vi "portinarisat_monitoreo.vi"() -> ()   [LabVIEW 2024]
uses:
  <vilib>/Instr/_visa.llb/VISA Configure Serial Port (Instr).vi
panel:
  out "?":dbl
  out "?":dbl
  out "?":dbl
  out "?":dbl
  out "?":dbl
  out "?":dbl
  out "?":dbl
  out "?":dbl
  out "?":dbl
  out "Trama original":string
  in  "Baudios":u32=9600
  in  "Puerto serial":refnum<visa-resource-name>
  in  "stop":bool
  out "Tiempo (s)":dbl
  out "Altitud":dbl
  out "Altitud (m)":dbl(slide) scale=0.0..500.0
  out "Altitud":i32(graph)
  out "Temperatura":i32(graph)
  out "Presión":i32(graph)
  out "CO2":i32(graph)
  out "CO2":dbl
  out "CO2 (ppm)":dbl(knob) scale=300.0..1000.0
  out "Temperatura":dbl
  out "Presiòn":dbl
  out "Velocidad":dbl
  out "G Eje Z":dbl(slide) caption="Eje Z" scale=-250.0..250.0
  out "G Eje Y":dbl(slide) caption="Eje Y" scale=-250.0..250.0
  out "G Eje X":dbl(slide) caption="Eje X" scale=-250.0..250.0
  out "CM Eje Z":dbl(slide) caption="Eje Z" scale=-60.0..60.0
  out "CM Eje Y":dbl(slide) caption="Eje Y" scale=-60.0..60.0
  out "CM Eje X":dbl(slide) caption="Eje X" scale=-60.0..60.0
  out "A Eje Z":dbl(slide) caption="Eje Z" scale=-20.0..20.0
  out "A Eje Y":dbl(slide) caption="Eje Y" scale=-20.0..20.0
  out "A Eje X":dbl(slide) caption="Eje X" scale=-20.0..20.0
  out "Velocidad (m/s)":dbl(knob) scale=-10.0..50.0
  out "Presión (kPa)":dbl(knob) scale=60.0..110.0
  out "Temperatura (°C)":dbl(slide) scale=-10.0..50.0
  # "Aceleración (m/s^2)"
  # "Campo magnético (µT)"
  # "Velocidad angular (°/s)"
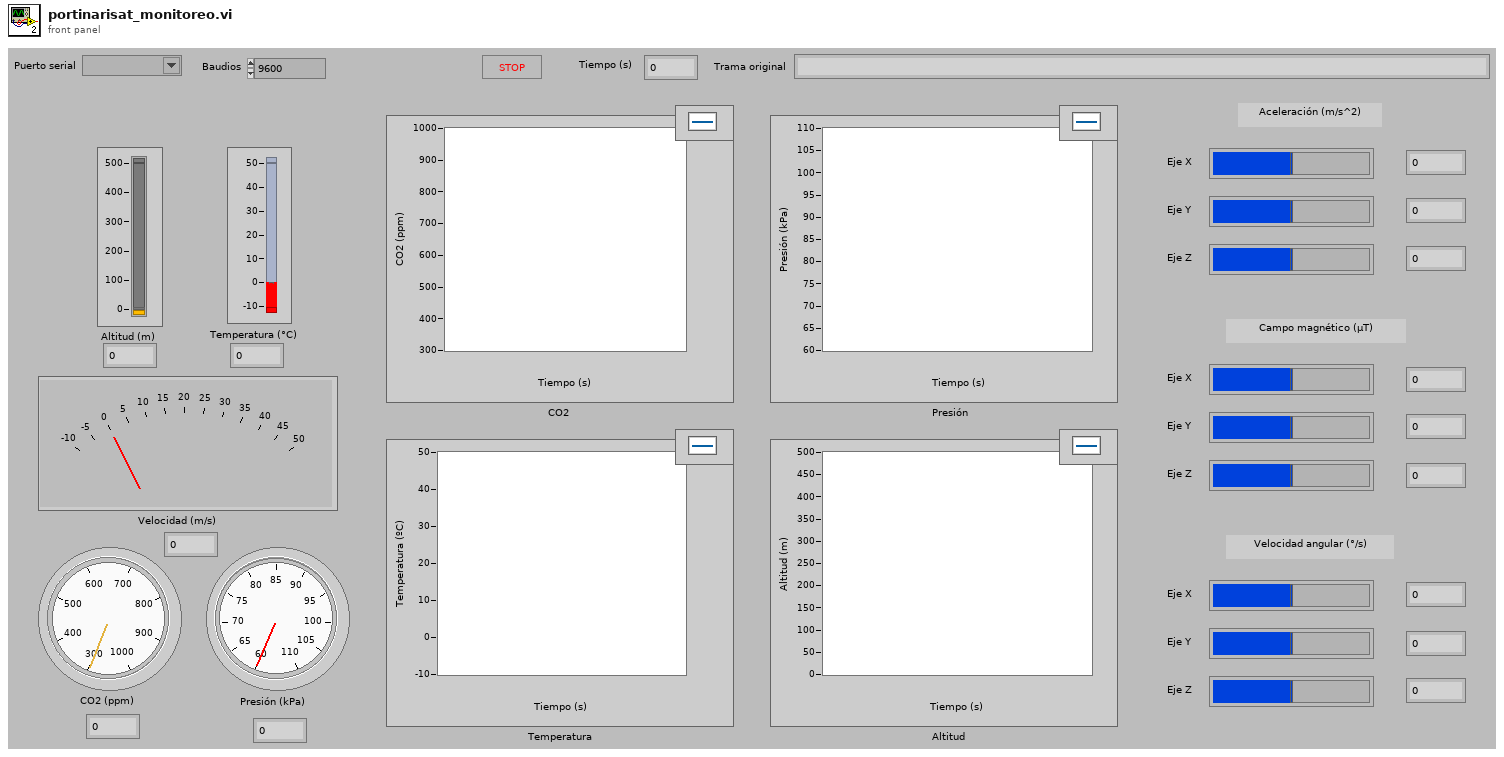
[diagram p1: front panel]
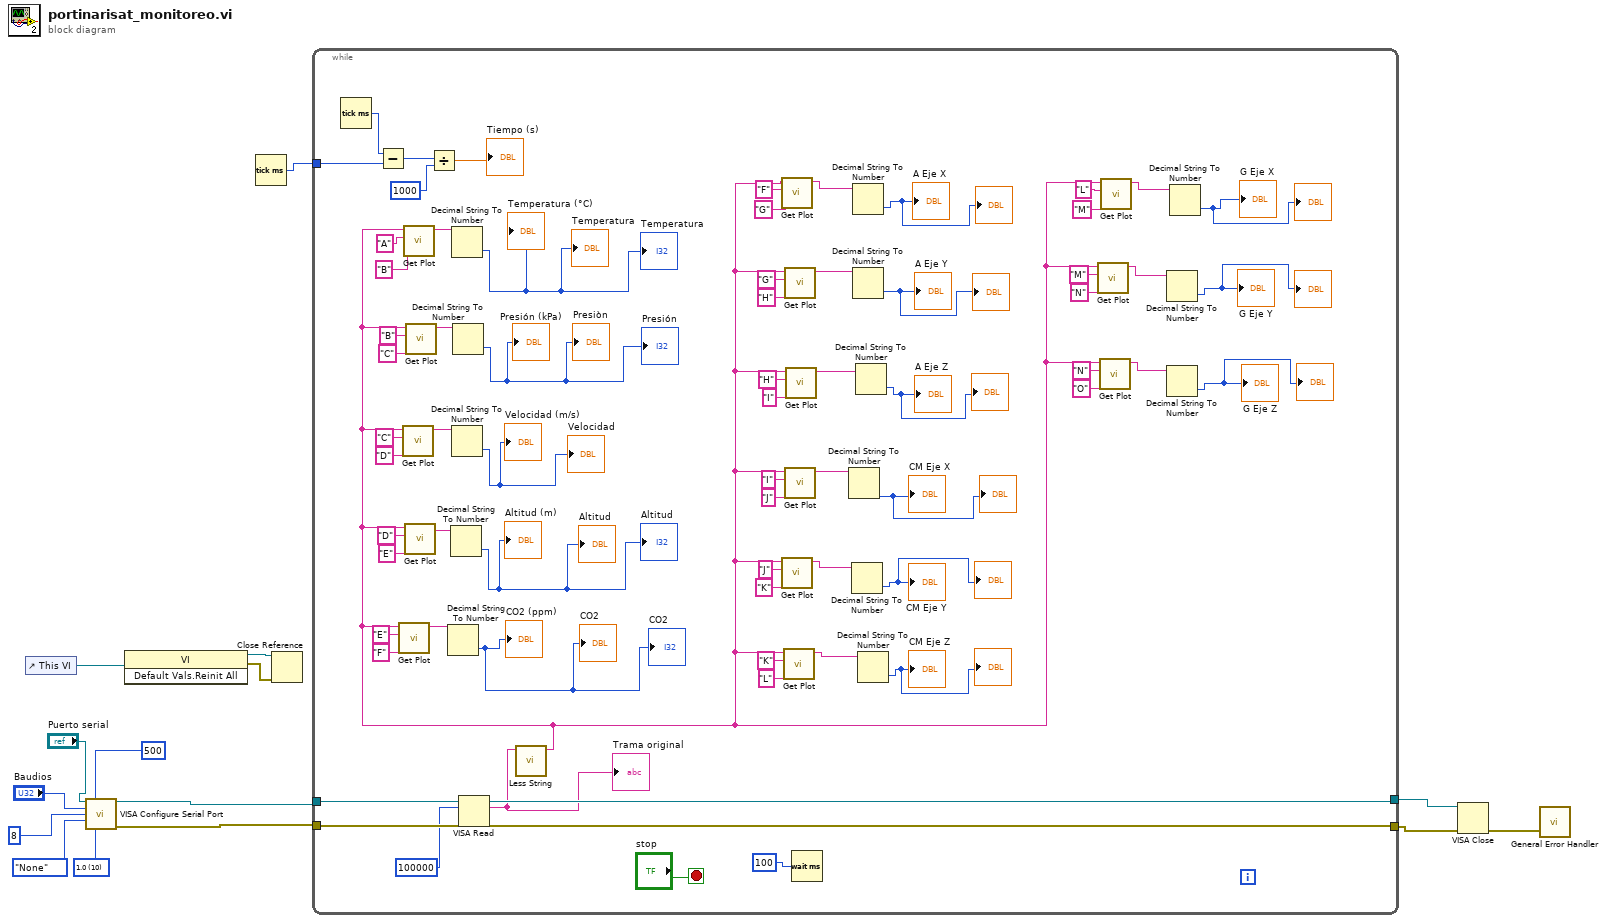
[diagram p0: block diagram]
diagram:
  w2 = u16 10 items=["1.0"=10, "1.5"=15, "2.0"=20] ("stop bits (10: 1 bit)")
  n1 = control-ref of="This VI"() -> (w8:refnum<vi>)
  n2 = call-poly "VISA Configure Serial Port"("VISA resource name"="Puerto serial", "timeout (10sec)"=u32 500, "baud rate (9600)"="Baudios", "data bits (8)"=u16 8, "parity (0:none)"=enum16{"None", "Odd", "Even", "Mark", "Space"}."None", "stop bits (10: 1 bit)"=w2) -> ("VISA resource name out"=w6:refnum<visa-resource-name>, "error out"=w5:errorcluster)  [unwired: 8 in]
  n3 = invoke class="VI" method="Default Vals.Reinit All"(reference=w8) -> (reference out=w9:refnum<vi>, error out=w7:errorcluster)  [unwired: 2 in, 1 out]
  n4 = Tick Count (ms)() -> (millisecond timer value=w11:u32)
  n5 = Close Reference(reference=w9, error in (no error)=w7) -> ()  [unwired: 1 out]
  n6 = while {
    tunnel: w6 -> [w28]
    tunnel: [w85] -> w13
    tunnel: [w83] -> w12
    tunnel: w11 -> [w33]
    tunnel: w5 -> [w29]
    stop <- "stop" stop-if-true
    n7 = Tick Count (ms)() -> (millisecond timer value=w34:u32)
    n8 = Subtract(x=w34, y=w33) -> (x-y=w32:u32)
    n9 = Divide(x=w32, y=u32 1000) -> (x/y=→"Tiempo (s)":dbl)
    n10 = VISA Read(VISA resource name=w28, byte count=u32 100000, error in (no error)=w29) -> (VISA resource name out=w85:refnum<visa-resource-name>, read buffer=w30:string, error out=w83:errorcluster)  [unwired: 1 out]
    "Trama original" <- w30
    n11 = call "Less String.vi"("Input String"=w30) -> ("Out String"=w60:string)  [unwired: 10 in]
    n12 = call "Get Plot.vi"("Stop"="F", "Start"="E", "Input String"=w60) -> ("Out String"=w47:string)  [unwired: 8 in]
    n13 = call "Get Plot.vi"("Stop"="D", "Start"="C", "Input String"=w60) -> ("Out String"=w50:string)  [unwired: 8 in]
    n14 = call "Get Plot.vi"("Stop"="B", "Start"="A", "Input String"=w60) -> ("Out String"=w53:string)  [unwired: 8 in]
    n15 = call "Get Plot.vi"("Stop"="E", "Start"="D", "Input String"=w60) -> ("Out String"=w49:string)  [unwired: 8 in]
    n16 = call "Get Plot.vi"("Stop"="C", "Start"="B", "Input String"=w60) -> ("Out String"=w52:string)  [unwired: 8 in]
    n17 = Decimal String To Number(string=w47) -> (number=→"CO2 (ppm)" →"CO2" →"CO2":i32)  [unwired: 2 in, 1 out]
    n18 = Decimal String To Number(string=w49) -> (number=→"Altitud" →"Altitud (m)" →"Altitud":i32)  [unwired: 2 in, 1 out]
    n19 = Decimal String To Number(string=w53) -> (number=→"Temperatura (°C)" →"Temperatura" →"Temperatura":i32)  [unwired: 2 in, 1 out]
    n20 = Decimal String To Number(string=w50) -> (number=→"Velocidad (m/s)" →"Velocidad":i32)  [unwired: 2 in, 1 out]
    n21 = Decimal String To Number(string=w52) -> (number=→"Presión (kPa)" →"Presiòn" →"Presión":i32)  [unwired: 2 in, 1 out]
    n22 = call "Get Plot.vi"("Stop"="G", "Start"="F", "Input String"=w60) -> ("Out String"=w45:string)  [unwired: 8 in]
    n23 = call "Get Plot.vi"("Stop"="K", "Start"="J", "Input String"=w60) -> ("Out String"=w41:string)  [unwired: 8 in]
    n24 = call "Get Plot.vi"("Stop"="L", "Start"="K", "Input String"=w60) -> ("Out String"=w40:string)  [unwired: 8 in]
    n25 = call "Get Plot.vi"("Stop"="H", "Start"="G", "Input String"=w60) -> ("Out String"=w44:string)  [unwired: 8 in]
    n26 = call "Get Plot.vi"("Stop"="J", "Start"="I", "Input String"=w60) -> ("Out String"=w42:string)  [unwired: 8 in]
    n27 = call "Get Plot.vi"("Stop"="I", "Start"="H", "Input String"=w60) -> ("Out String"=w43:string)  [unwired: 8 in]
    n28 = Wait (ms)(milliseconds to wait=u32 100) -> ()  [unwired: 1 out]
    n29 = Decimal String To Number(string=w42) -> (number=→"CM Eje X" →"?":i32)  [unwired: 2 in, 1 out]
    n30 = Decimal String To Number(string=w41) -> (number=→"CM Eje Y" →"?":i32)  [unwired: 2 in, 1 out]
    n31 = Decimal String To Number(string=w45) -> (number=→"A Eje X" →"?":i32)  [unwired: 2 in, 1 out]
    n32 = Decimal String To Number(string=w44) -> (number=→"A Eje Y" →"?":i32)  [unwired: 2 in, 1 out]
    n33 = Decimal String To Number(string=w43) -> (number=→"A Eje Z" →"?":i32)  [unwired: 2 in, 1 out]
    n34 = Decimal String To Number(string=w40) -> (number=→"CM Eje Z" →"?":i32)  [unwired: 2 in, 1 out]
    n35 = call "Get Plot.vi"("Stop"="N", "Start"="M", "Input String"=w60) -> ("Out String"=w38:string)  [unwired: 8 in]
    n36 = call "Get Plot.vi"("Stop"="O", "Start"="N", "Input String"=w60) -> ("Out String"=w37:string)  [unwired: 8 in]
    n37 = call "Get Plot.vi"("Stop"="M", "Start"="L", "Input String"=w60) -> ("Out String"=w39:string)  [unwired: 8 in]
    n38 = Decimal String To Number(string=w38) -> (number=→"G Eje Y" →"?":i32)  [unwired: 2 in, 1 out]
    n39 = Decimal String To Number(string=w37) -> (number=→"G Eje Z" →"?":i32)  [unwired: 2 in, 1 out]
    n40 = Decimal String To Number(string=w39) -> (number=→"G Eje X" →"?":i32)  [unwired: 2 in, 1 out]
  }
  n41 = VISA Close(VISA resource name=w13, error in (no error)=w12) -> (error out=w10:errorcluster)
  n42 = call <vilib>:"General Error Handler.vi"("error in (no error)"=w10) -> ()  [unwired: 10 in, 5 out]
